vi "Remove duplicated LPTH.vi"(11 "items":string[](array[string])) -> (1 "Filenum":i32[](array[numeric]), 2 "Items out":string[](array[string]))   [LabVIEW 2017, in "Palette Menu.lvlib"]
uses:
  <vilib>/Palette API/Palette Menu/Palette Menu.lvlib
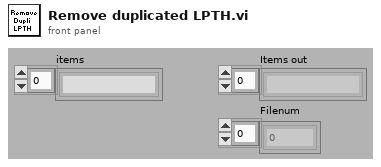
[diagram p1: front panel]
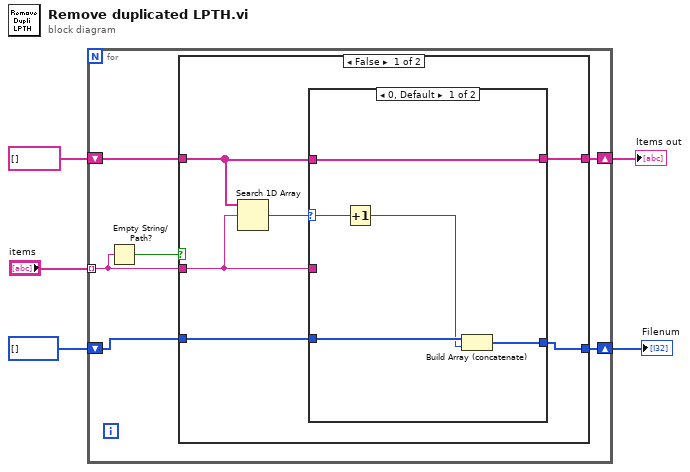
[diagram p0: block diagram]
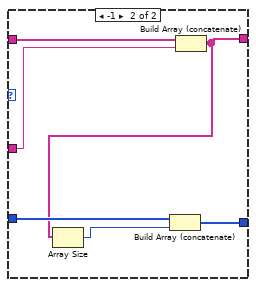
[diagram p2: hidden frame]
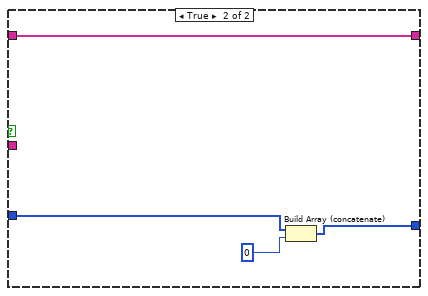
[diagram p3: hidden frame]
diagram:
  n1 = for {
    tunnel: "items" -> [w7] mode=indexing
    shift-right: [w8] -> w4
    shift-left: i32[] [] -> [w9]
    shift-right: [w10] -> w1
    shift-left: string[] [] ("items") -> [w11]
    n2 = Empty String/Path?(string/path=w7) -> (empty?=w6:bool)
    n3 = case shown="False" w6 {
      tunnel: w11 -> [w16 w32]
      tunnel: [w15 w32] -> w10
      tunnel: w9 -> [w14 w31]
      tunnel: [w13 w30] -> w8
      tunnel: w7 -> [w12 _]
      frame False {
        n4 = Search 1D Array(1D array=w16, element=w12) -> (index of element=w17:i32)  [unwired: 1 out]
        n5 = case shown="0, Default" w17 {
          selector: w17 -> [w19 _]
          tunnel: w12 -> [_ w27]
          tunnel: w16 -> [w22 w28]
          tunnel: [w22 w24] -> w15
          tunnel: w14 -> [w21 w25]
          tunnel: [w20 w26] -> w13
          frame 0, Default {
            n6 = Increment(x=w19) -> (x+1=w18:i32)
            n7 = Build Array (concatenate)(w21, w18) -> (w20:i32[])
          }
          frame -1 {
            n8 = Build Array (concatenate)(w28, w27) -> (w24:string[])
            n9 = Array Size(array=w24) -> (size(s)=w23:i32)
            n10 = Build Array (concatenate)(w25, w23) -> (w26:i32[])
          }
        }
      }
      frame True {
        n11 = Build Array (concatenate)(w31, 0) -> (w30:i32[])
      }
    }
  }
  "Filenum" <- w4
  "Items out" <- w1
